vi "shutdown.vi"(7 "references":T1, 8 "error in (no error)":errorcluster, 11 "wait_ms":i32) -> (0 "error out":errorcluster, 3 "unfinished":i32)   [LabVIEW 2015, in "lv-recipe-machine.lvlib"]
uses:
  lv-recipe-machine.lvlib
  _controls/references.ctl
  _controls/input.ctl
  _controls/input_command.ctl
  _controls/output.ctl
  _controls/data.ctl
  _controls/configuration.ctl
  _controls/recipe_data.ctl
  _controls/mode.ctl
  _controls/manual_state.ctl
  _controls/automatic_state.ctl
  _controls/recipe_step.ctl
  <userlib>/antonio-alexander/lv-waitgroup/public/_controls/api_waitgroup.ctl
  _controls/change.ctl
  _controls/status.ctl
  <userlib>/antonio-alexander/lv-waitgroup/lv-waitgroup.lvlib
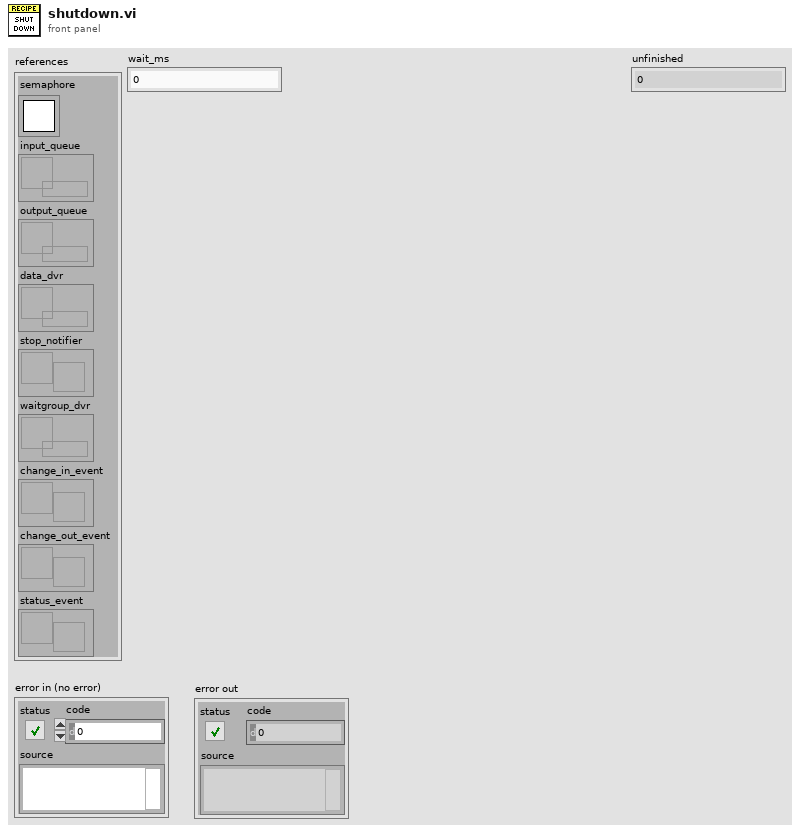
[diagram p1: front panel]
types:
  T1 = typedef "lv-recipe-machine.lvlib/references.ctl" = cluster{"semaphore":T2, "input_queue":refnum<queue>, "output_queue":refnum<queue>, "data_dvr":refnum<data-value>, "stop_notifier":refnum<notifier>, "waitgroup_dvr":refnum<data-value>, "change_in_event":refnum<user-event>, "change_out_event":refnum<user-event>, "status_event":refnum<user-event>}
  T2 = typedef "Semaphore RefNum" = refnum<k1>
  T3 = typedef "lv-waitgroup.lvlib/api_waitgroup.ctl" = cluster{"waitgroups":refnum<data-value>, "waitgroup":string}
  T4 = typedef "lv-recipe-machine.lvlib/data.ctl" = cluster{"configuration":T5, "working":cluster{"recipe_data":T6, "api_waitgroup":T3}}
  T5 = typedef "lv-recipe-machine.lvlib/configuration.ctl" = cluster{"max_processes":i32}
  T6 = typedef "lv-recipe-machine.lvlib/recipe_data.ctl" = cluster{"mode":T7, "manual_state":T8, "automatic_state":T9, "previous_automatic_state":T9, "error":errorcluster, "manual":cluster{"step_action":string, "data":variant, "actions":variant}, "automatic":cluster{"data":variant, "steps":variant, "criteria":variant, "transition":string, "index":i32, "recipe []":T10[]}}
  T7 = typedef "lv-recipe-machine.lvlib/mode.ctl" = enum16{"<mode>", "manual", "automatic", "<null>"}
  T8 = typedef "lv-recipe-machine.lvlib/manual_state.ctl" = enum16{"<manual_state>", "failed", "action", "running", "idle", "<null>"}
  T9 = typedef "lv-recipe-machine.lvlib/automatic_state.ctl" = enum16{"<automatic_state>", "failed", "idle", "running", "paused", "transition", "stopped", "<null>"}
  T10 = typedef "lv-recipe-machine.lvlib/recipe_step.ctl" = cluster{"step":string, "data":variant}
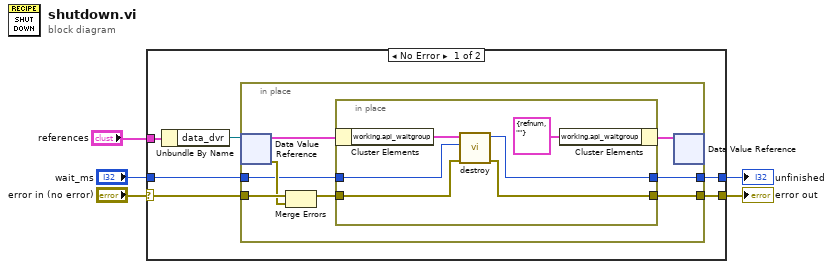
[diagram p0: block diagram]
diagram:
  n1 = case shown="No Error" "error in (no error)" {
    selector: "error in (no error)" -> [w8 w26]
    tunnel: [w10 w26] -> w4
    tunnel: "references" -> [w9 _]
    tunnel: [w7 _] -> w2
    tunnel: "wait_ms" -> [w6 _]
    frame No Error {
      n2 = Unbundle By Name(w9) -> ("data_dvr"=w11:refnum<data-value>)
      n3 = in-place {
        in-place-border: [w14] -> w10
        in-place-border: w8 -> [w19]
        in-place-border: [w13] -> w7
        in-place-border: w6 -> [w12]
        n4 = in-place-dvr #1(w11) -> (w17:T4, w18:errorcluster)
        n5 = Merge Errors(w19, w18) -> (w16:errorcluster)
        n6 = in-place {
          in-place-border: w16 -> [w24]
          in-place-border: [w22] -> w14
          in-place-border: [w21] -> w13
          in-place-border: w12 -> [w20]
          n7 = in-place-cluster #2(w17) -> ("working.api_waitgroup"=w25:T3)
          n8 = call <userlib>:"destroy.vi"("error in (no error)"=w24, "wait_ms"=w20, "waitgroup"=w25) -> ("error out"=w22:errorcluster, "unfinished"=w21:i32)  [unwired: 7 in]
          n9 = in-place-cluster #2("working.api_waitgroup"=T3 {"waitgroups"=refnum, "waitgroup"=""}) -> (w15:T4)
        }
        n10 = in-place-dvr #1(w15) -> ()  [unwired: 2 out]
      }
    }
    frame Error {
    }
  }
  "error out" <- w4
  "unfinished" <- w2
